vi "read_write path.vi"(10 "path in":path, 11 "type(read)":enum16{"read", "write"}(ring)) -> (2 "path out":path, 3 "out":string)   [LabVIEW 2018]
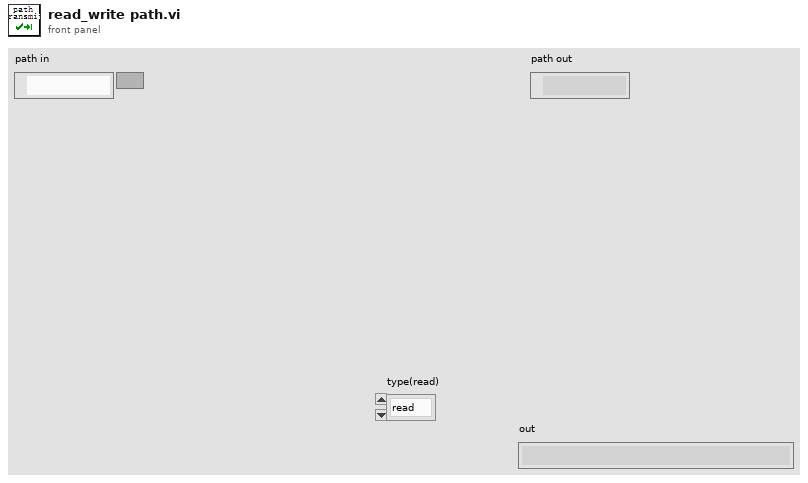
[diagram p1: front panel]
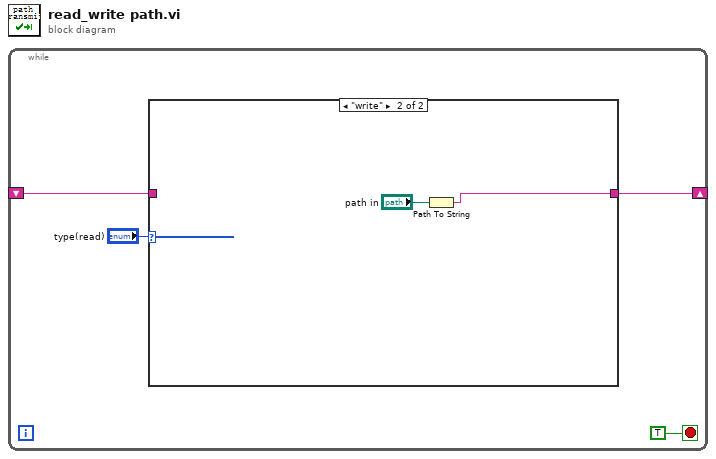
[diagram p0: block diagram]
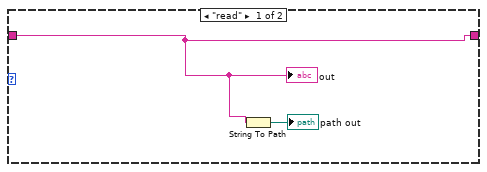
[diagram p2: hidden frame]
diagram:
  n1 = while {
    shift-right: [w3] -> _
    shift-left: _ -> [w2]
    stop <- TRUE stop-if-true
    n2 = case shown="\"write\"" "type(read)" {
      tunnel: [w6 w8] -> w3
      tunnel: w2 -> [w6 _]
      frame "read" {
        n3 = String To Path(string=w6) -> (path=→"path out":path)
        "out" <- w6
      }
      frame "write" {
        n4 = Path To String(path="path in") -> (string=w8:string)
      }
    }
  }
